vi "daq_light_sensors.vi"(1 "Timeout":i32) -> (0 "FIFO_timeout":bool)   [LabVIEW 2018]
uses:
  <vilib>/rvi/eio/common/nirviEmuTemplateMethod_errors.vi
  <vilib>/rvi/DataTransferAndStorage/Container/Common/niFpgaContainerExecOnDevCompGetState.vi
  <vilib>/rvi/Emulation/niFpgaEmulationIsFPGAContextNoSignature.vi
  <vilib>/rvi/Emulation/niFpgaSctlEmulationGetInTimedLoop.vi
  <vilib>/rvi/errors/niFpgaSetErrorForExecOnDevCompSimple.vi
  <vilib>/rvi/eio/common/nirviEmuReportErrorAndStop.vi
  <vilib>/rvi/DataTransferAndStorage/Container/Common/niFpgaContainerGetUniqueNameForEmu.vi
  <vilib>/rvi/FIFO/Fifo_Resource/nirvififoEmulationSetSize.vi
  <vilib>/rvi/FIFO/Fifo_Resource/nirviFifoEmulationQueueMgr.vi
  <instcachedir>/0/nirviFifoEmulationQueueMgr_E5CAEC123FF24DC58D834DCA3CDAA9B5.lvgen/nirviFifoEmulationQueueMgr_E5CAEC123FF24DC58D834DCA3CDAA9B5_001.vi
  <vilib>/rvi/FIFO/Fifo_Resource/nirvififoEmulationDetermineInputValidOut.vi
  <vilib>/rvi/FIFO/Fifo_Resource/nirvififoEmulationCreateLock.vi
  <vilib>/rvi/Emulation/niFpgaProcessEmulError.vi
  <vilib>/rvi/FIFO/Fifo_Resource/nirvififoEmulationObtainLock.vi
  <vilib>/rvi/FIFO/Fifo_Resource/nirvififoEmulationReleaseLock.vi
  <vilib>/rvi/occurrence/nirviWaitOnOccurrenceBase.vi
  <vilib>/rvi/errors/nirviReportUnexpectedCaseInternalError.vi
  <vilib>/rvi/errors/nirviReportUnexpectedCaseInternalError (U32).vi
  <vilib>/Utility/error.llb/Clear Errors.vi
  <vilib>/rvi/interface/RandomDataEmulation/niFpgaRandomDataHandleErrors.vi
  <vilib>/eio/EIONode/EIONode.xnode
  <vilib>/rvi/DataTransferAndStorage/Container/XNode/niFpgaContainer.xnode
  <vilib>/rvi/FIFO/Fifo_Resource/niFpgaFifoEmulationRefIn.vi
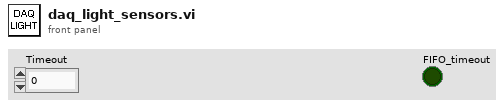
[diagram p1: front panel]
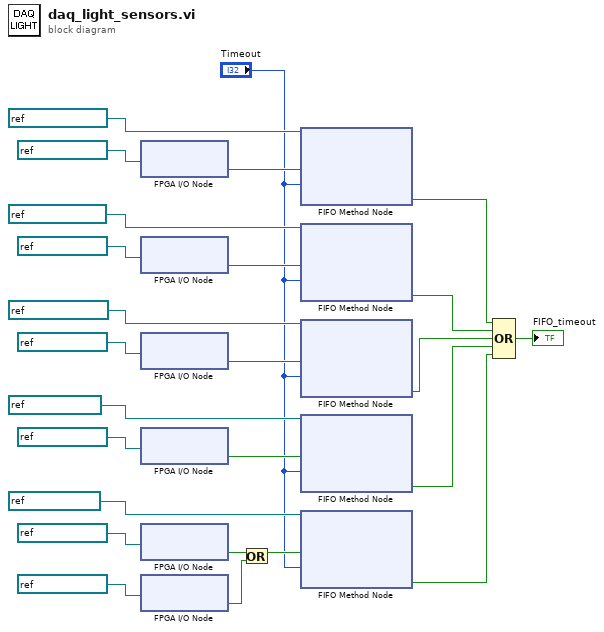
[diagram p0: block diagram]
diagram:
  n1 = xnode "FPGA I/O Node"("FPGA I/O In"=refnum<k21> "Mod2/DIO0") -> ("I/O Item"=w24:bool)  [unwired: 1 out]
  n2 = xnode "FPGA I/O Node"("FPGA I/O In"=refnum<k21> "Mod2/DIO1") -> ("I/O Item"=w21:bool)  [unwired: 1 out]
  n3 = xnode "FPGA I/O Node"("FPGA I/O In"=refnum<k21> "Mod2/DIO2") -> ("I/O Item"=w18:bool)  [unwired: 1 out]
  n4 = xnode "FPGA I/O Node"("FPGA I/O In"=refnum<k21> "Mod2/DIO5") -> ("I/O Item"=w15:bool)  [unwired: 1 out]
  n5 = xnode "FPGA I/O Node"("FPGA I/O In"=refnum<k21> "Mod2/DIO3") -> ("I/O Item"=w12:bool)  [unwired: 1 out]
  n6 = xnode "FPGA I/O Node"("FPGA I/O In"=refnum<k21> "Mod2/DIO4") -> ("I/O Item"=w8:bool)  [unwired: 1 out]
  n7 = Or(x=w12, y=w8) -> (x .or. y?=w9:bool)
  n8 = xnode ("FIFO Method Node")("Element"=w24, "Timeout"="Timeout", "FIFO In"=refnum<k21> "FIFO_light_FR") -> ("Timed Out?"=w6:bool)  [unwired: 1 out]
  n9 = xnode ("FIFO Method Node")("Element"=w21, "Timeout"="Timeout", "FIFO In"=refnum<k21> "FIFO_light_FL") -> ("Timed Out?"=w5:bool)  [unwired: 1 out]
  n10 = xnode ("FIFO Method Node")("Element"=w18, "Timeout"="Timeout", "FIFO In"=refnum<k21> "FIFO_light_BR") -> ("Timed Out?"=w2:bool)  [unwired: 1 out]
  n11 = xnode ("FIFO Method Node")("Element"=w15, "Timeout"="Timeout", "FIFO In"=refnum<k21> "FIFO_laser_R") -> ("Timed Out?"=w3:bool)  [unwired: 1 out]
  n12 = xnode ("FIFO Method Node")("Element"=w9, "Timeout"="Timeout", "FIFO In"=refnum<k21> "FIFO_laser_L") -> ("Timed Out?"=w4:bool)  [unwired: 1 out]
  n13 = Compound Arithmetic op=OR(w6, w5, w2, w3, w4) -> (→"FIFO_timeout":bool)
